vi "Get Request Type.vi"(8 "error in (no error)":errorcluster, 11 "GetInputKindList in":refnum<class "GetInputKindList.lvclass">) -> (0 "error out":errorcluster, 2 "Request Type":string, 3 "GetInputKindList out":refnum<class "GetInputKindList.lvclass">)   [LabVIEW 2020, in "obs-websocket.lvlib" / "GetInputKindList.lvclass"]
uses:
  GetInputKindList.lvclass
  GetInputKindList.lvclass/GetInputKindList.ctl
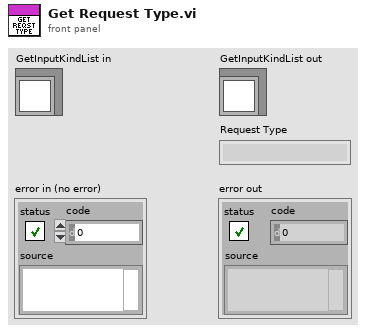
[diagram p1: front panel]
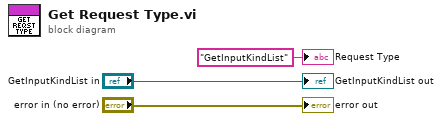
[diagram p0: block diagram]
diagram:
  "error out" <- "error in (no error)"
  "GetInputKindList out" <- "GetInputKindList in"
  "Request Type" <- "GetInputKindList" ("Request Type")
